vi "Firebase.vi"() -> ()   [LabVIEW 2020]
uses:
  <vilib>/httpClient/PUTBuffer.vi
  <vilib>/httpClient/LabVIEWHTTPClient.lvlib
panel:
  in  "LED":dbl(slide) scale=0.0..255.0
  in  "LED Control":bool
  in  "servo":dbl(slide) scale=0.0..180.0
  in  "Servo control":bool
  out "LDR":dbl(slide) scale=0.0..10.0
  out "Image Out":T1(plugin-control)
  out "Ultrasonic distance":dbl
  out "Radar":picture
  out "Recieve":string
  out "Send":string
  out "LDR":dbl
  out "ULTRA SONIC":dbl
  out "SERVO":dbl
  in  "stop":bool
  in  "Speed":dbl(slide) scale=0.0..255.0
  in  "Left":bool
  in  "Right":bool
  in  "Down":bool
  in  "Up":bool
  out "concatenated string 2":string
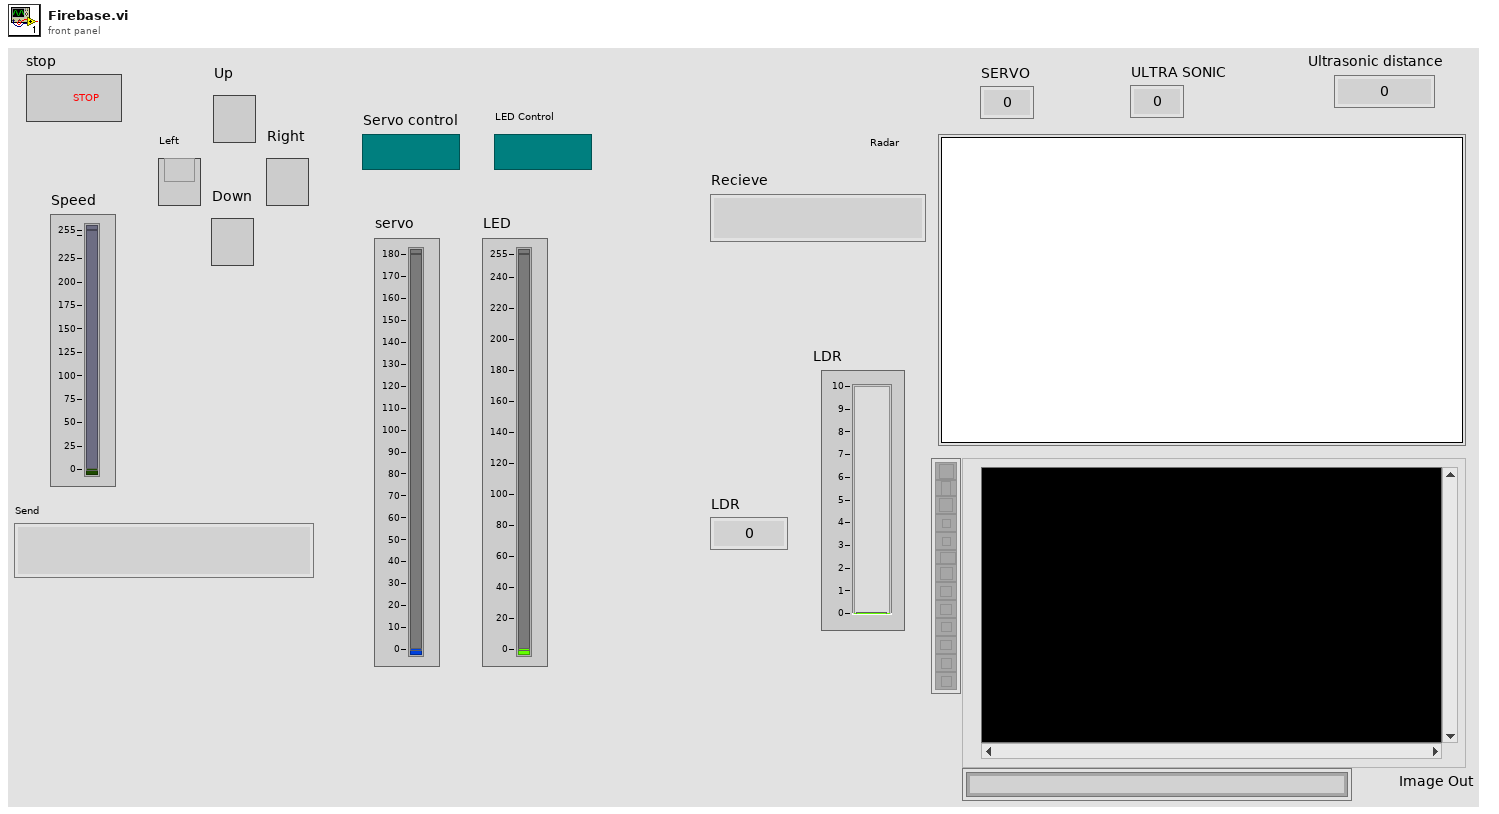
[diagram p1: front panel]
types:
  T1 = typedef "IMAQ Image.ctl" = refnum<image>
  T2 = typedef "LabVIEWHTTPClient.lvlib/ClientHandle.ctl" = refnum<k1>
  T3 = cluster{"maximum":dbl, "minimum":dbl, "clip to min":bool, "log?(F)":bool, "grid color":u32, "plot color":u32, "fmt and prec":cluster{"format":enum8{"Decimal", "Scientific", "Engineering", "Binary", "Octal", "Hex"}, "precision":u8}, "visible section":u16}
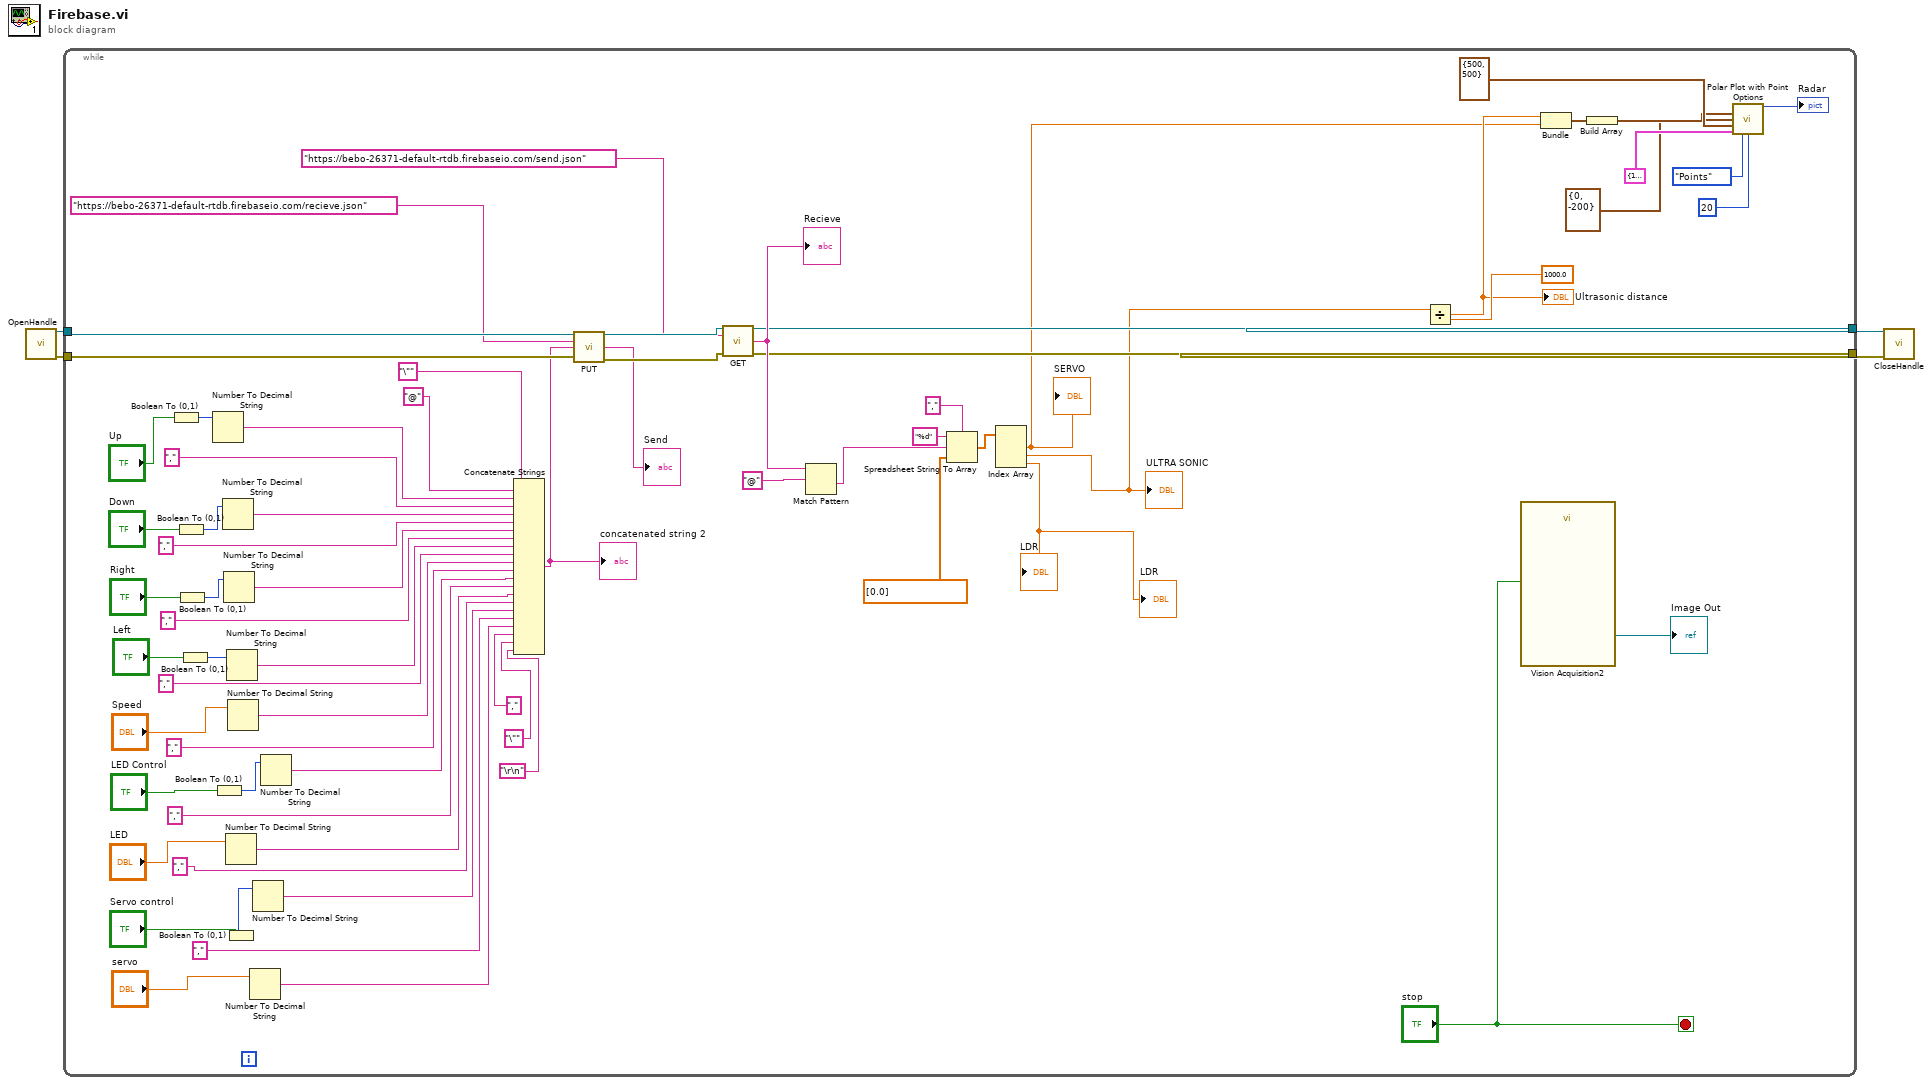
[diagram p0: block diagram]
diagram:
  n1 = call <vilib>:"OpenHandle.vi"() -> ("client handle out"=w4:T2, "error out"=w3:errorcluster)  [unwired: 14 in]
  n2 = while {
    tunnel: w4 -> [w49]
    tunnel: w3 -> [w50]
    tunnel: [w42] -> w2
    tunnel: [w41] -> w1
    stop <- "stop" stop-if-true
    n3 = Boolean To (0,1)(Boolean="Up") -> (0, 1=w64:i16)
    n4 = Boolean To (0,1)(Boolean="Down") -> (0, 1=w60:i16)
    n5 = Boolean To (0,1)(Boolean="Right") -> (0, 1=w59:i16)
    n6 = Boolean To (0,1)(Boolean="Left") -> (0, 1=w58:i16)
    n7 = Number To Decimal String(number=w64) -> (decimal integer string=w73:string)  [unwired: 1 in]
    n8 = Boolean To (0,1)(Boolean="LED Control") -> (0, 1=w19:i16)
    n9 = Number To Decimal String(number=w60) -> (decimal integer string=w71:string)  [unwired: 1 in]
    n10 = Number To Decimal String(number=w59) -> (decimal integer string=w69:string)  [unwired: 1 in]
    n11 = Number To Decimal String(number="LED") -> (decimal integer string=w12:string)  [unwired: 1 in]
    n12 = Boolean To (0,1)(Boolean="Servo control") -> (0, 1=w22:i16)
    n13 = Number To Decimal String(number=w58) -> (decimal integer string=w67:string)  [unwired: 1 in]
    n14 = Number To Decimal String(number="Speed") -> (decimal integer string=w16:string)  [unwired: 1 in]
    n15 = Number To Decimal String(number="servo") -> (decimal integer string=w8:string)  [unwired: 1 in]
    n16 = Number To Decimal String(number=w22) -> (decimal integer string=w10:string)  [unwired: 1 in]
    n17 = Number To Decimal String(number=w19) -> (decimal integer string=w14:string)  [unwired: 1 in]
    n18 = Concatenate Strings("\"" ("string"), "@" ("string"), w73, "," ("string"), w71, "," ("string"), w69, "," ("string"), w67, "," ("string"), w16, "," ("string"), w14, "," ("string"), w12, "," ("string"), w10, "," ("string"), w8, "," ("string"), "\"" ("string"), "\r\n") -> (w40:string)
    "concatenated string 2" <- w40
    n19 = call-poly <vilib>:"PUT.vi"("client handle"=w49, "url"="https://bebo-26371-default-rtdb.firebaseio.com/recieve.json", "buffer"=w40, "error in (no error)"=w50) -> ("client handle out"=w47:T2, "body"=→"Send":string, "error out"=w46:errorcluster)  [unwired: 8 in, 1 out]
    n20 = call <vilib>:"GET.vi"("client handle"=w47, "url"="https://bebo-26371-default-rtdb.firebaseio.com/send.json", "error in (no error)"=w46) -> ("client handle out"=w42:T2, "body"=w44:string, "error out"=w41:errorcluster)  [unwired: 9 in, 1 out]
    "Recieve" <- w44
    n21 = Match Pattern(string=w44, regular expression="@") -> (after substring=w51:string)  [unwired: 1 in, 3 out]
    n22 = Spreadsheet String To Array(delimiter (Tab)=",", format string="%d", spreadsheet string=w51, array type (2D Dbl)=dbl[] [0.0]) -> (array=w53:dbl[])
    n23 = Index Array(array=w53) -> (element #1=w23:dbl, element #2=w24:dbl, element #3=→"LDR" →"LDR":dbl)  [unwired: 3 in]
    "SERVO" <- w23
    "ULTRA SONIC" <- w24
    n24 = Divide(x=w24, y=1000.0) -> (x/y=w31:dbl)
    "Ultrasonic distance" <- w31
    n25 = call "Vision Acquisition2"("Stop (F)"="stop") -> ("Image Out"=→"Image Out":T1)  [unwired: 24 in, 2 out]
    n26 = Bundle "Bundle"(w31, w23) -> (w37:cluster{dbl, dbl})  [unwired: 1 in]
    n27 = Build Array "Build Array"(w37) -> (w27:cluster{dbl, dbl}[])
    n28 = call <vilib>:"Polar Plot with Point Options.vi"("data array [mag, phase (deg)]"=w27, "top left point(0, 0)"=cluster{"x":i16, "y":i16} {"x"=0, "y"=-200}, "dimensions (w,h)"=cluster{"width":i16, "height":i16} {"width"=500, "height"=500}, "polar attributes"=T3 {"maximum"=10.0, "minimum"=0.0, "clip to min"=FALSE, "log?(F)"=FALSE, "grid color"=131586, "plot color"=6618880, "fmt and prec"={"format"=enum."Decimal", "precision"=2}, "visible section"=4}, "Lines/Points"=enum16{"Lines", "Points"}."Points", "Size"=u16 20) -> ("new picture"=→"Radar":picture)  [unwired: 9 in]
  }
  n29 = call <vilib>:"CloseHandle.vi"("client handle"=w2, "error in (no error)"=w1) -> ()  [unwired: 13 in, 1 out]
